vi "Motor Initial 2(SubVI).vi"(11 "Cluster in 2":T1 {"Motor Step" items=["1 deg"=1, "3 deg"=3, "5 deg"=5, "10 deg"=10]; "Motor Range" items=["40 deg"=40, "360 deg"=360, "180 deg"=180]; "Mode" items=["Create", "Delete", "Select"]; "IF Bandwidth" format="%.3p"; "Span Freq" format="%.3p"; "Center Freq" format="%.3p"; "Power Level" format="%.2p"}) -> (2 "Locat":dbl caption="Current Location" format="%#.1f deg.", 3 "Cluster in 3":T1 {"Motor Step" items=["1 deg"=1, "3 deg"=3, "5 deg"=5, "10 deg"=10]; "Motor Range" items=["40 deg"=40, "360 deg"=360, "180 deg"=180]; "Mode" items=["Create", "Delete", "Select"]; "IF Bandwidth" format="%.3p"; "Span Freq" format="%.3p"; "Center Freq" format="%.3p"; "Power Level" format="%.2p"})   [LabVIEW 2020]
uses:
  Chamber_2018/ControlCluster.ctl
  D:/BWant RT/BWant_RT.lvlibp/Control Function.ctl
  D:/BWant RT/BWant_RT.lvlibp
panel:
  in  "Stop":bool
  out "[ALM-A]":bool
  in  "Mode":enum16{"INC", "ABS"}(ring)=enum."ABS"
  out "[READY]":bool
  # "Hz"
  # "Hz"
  # "Hz"
  # "dBm"
  # "Hz"
  # "Hz"
  # "Hz"
  # "dBm"
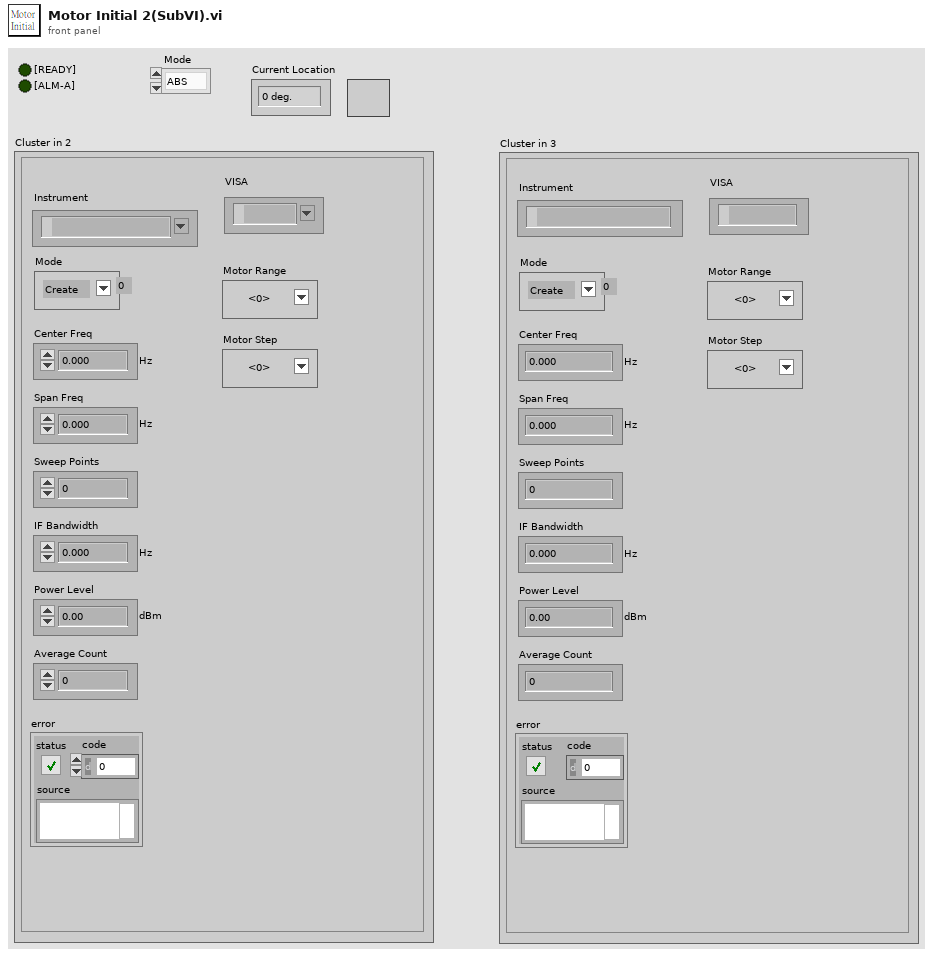
[diagram p1: front panel]
types:
  T1 = typedef "ControlCluster.ctl" = cluster{"Power Level":dbl, "Center Freq":dbl, "Span Freq":dbl, "Sweep Points":u32, "IF Bandwidth":dbl, "Average Count":i32, "error":errorcluster, "Instrument":refnum<visa-resource-name>, "Mode":u16, "Motor Range":u16, "Motor Step":u16, "VISA":refnum<visa-resource-name>}
  T2 = typedef "BWant_RT.lvlibp/Control Function.ctl" = enum16{"Idle", "Initial", "Close", "Check State", "ALM Reset", "ALM Inf", "Preset Home", "Pst_Value", "Speed", "Start-slope", "End-slpoe", "Read Pst", "GO Home", "Move", "Stop", "Limit mode", "MLU", "MLL", "Direction"}
  T3 = cluster{"[MOVE]":bool, "[READY]":bool, "[ALM-A]":bool}
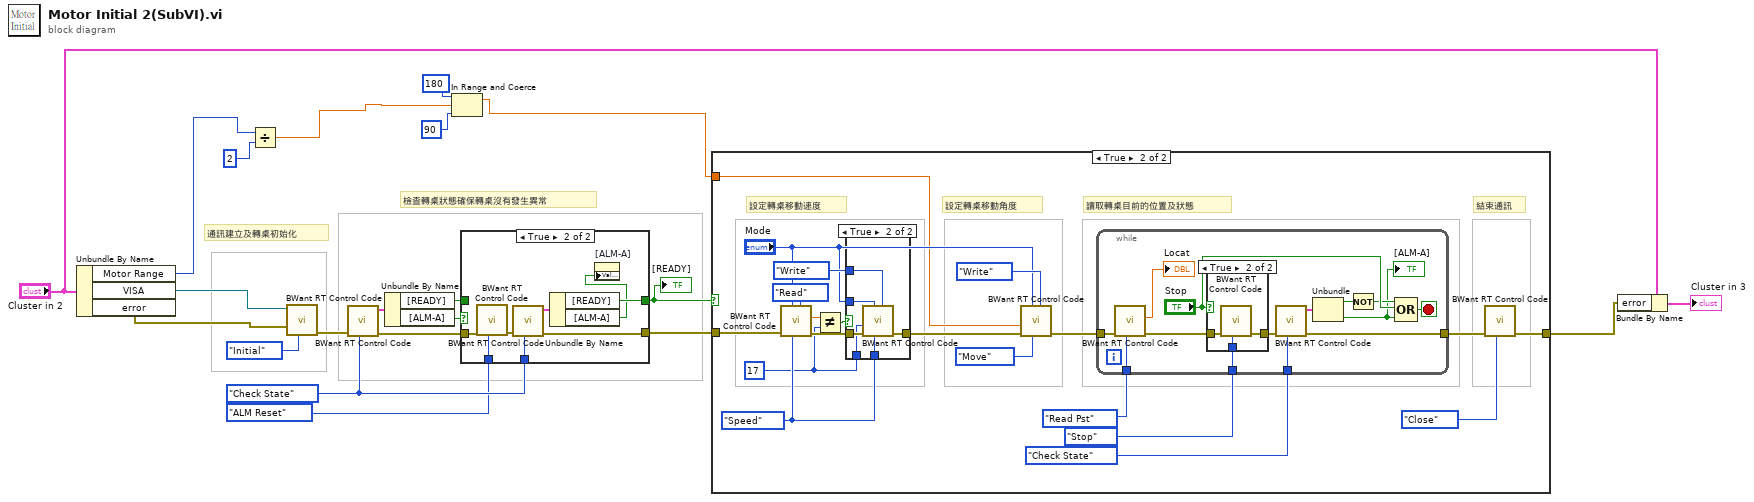
[diagram p0: block diagram]
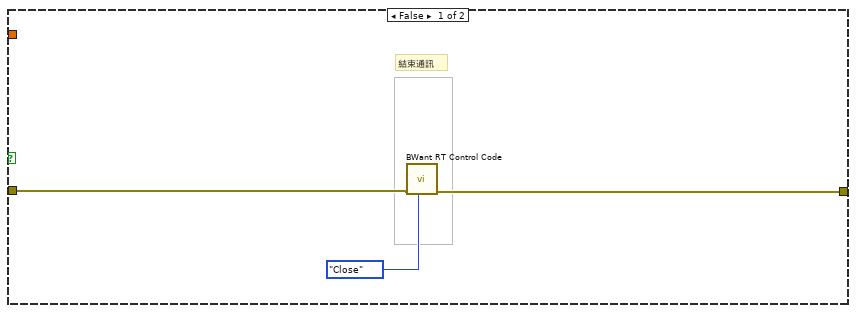
[diagram p2: hidden frame]
diagram:
  w13 = Control_Function."Check State" ("Fn")
  # "檢查轉桌狀態確保轉桌沒有發生異常"
  # "通訊建立及轉桌初始化"
  n1 = Unbundle By Name("Cluster in 2") -> ("Motor Range"=w9:u16, "VISA"=w11:refnum<visa-resource-name>, "error"=w10:errorcluster)
  n2 = Divide(x=w9, y=2) -> (x/y=w2:dbl)
  n3 = call "BWant RT Control Code.vi"("Fn"=Control_Function."Initial", "error in"=w10, "ComPort"=w11) -> ("error out"=w18:errorcluster)  [unwired: 5 in, 3 out]
  n4 = call "BWant RT Control Code.vi"("Fn"=w13, "error in"=w18) -> ("error out"=w20:errorcluster, "State"=w19:T3)  [unwired: 6 in, 2 out]
  n5 = Unbundle By Name(w19) -> ("[READY]"=w17:bool, "[ALM-A]"=w21:bool)
  n6 = In Range and Coerce(upper limit=180, x=w2, lower limit=90) -> (coerced(x)=w1:dbl)  [unwired: 1 out]
  n7 = case shown="True" w21 {
    tunnel: [w23 w29] -> w16
    tunnel: w20 -> [w23 w25]
    tunnel: Control_Function."ALM Reset" ("Fn") -> [_ w31]
    tunnel: w13 -> [_ w28]
    tunnel: [w22 w26] -> w15
    tunnel: w17 -> [w22 _]
    frame False {
    }
    frame True {
      n8 = call "BWant RT Control Code.vi"("Fn"=w31, "error in"=w25) -> ("error out"=w30:errorcluster)  [unwired: 6 in, 3 out]
      n9 = call "BWant RT Control Code.vi"("Fn"=w28, "error in"=w30) -> ("error out"=w29:errorcluster, "State"=w27:T3)  [unwired: 6 in, 2 out]
      n10 = Unbundle By Name(w27) -> ("[READY]"=w26:bool, "[ALM-A]"=w24:bool)
      n11 = property on="[ALM-A]" class="Bool (strict)"("Value"=w24) -> ()  [unwired: 2 in, 2 out]
    }
  }
  "[READY]" <- w15
  n12 = case shown="True" w15 {
    tunnel: w16 -> [w34 w54]
    tunnel: [w33 w44] -> w5
    tunnel: w1 -> [_ w36]
    frame False {
      # "結束通訊"
      n13 = call "BWant RT Control Code.vi"("Fn"=Control_Function."Close", "error in"=w34) -> ("error out"=w33:errorcluster)  [unwired: 6 in, 3 out]
    }
    frame True {
      w35 = 17
      w42 = Control_Function."Speed" ("Fn")
      # "結束通訊"
      # "讀取轉桌目前的位置及狀態"
      # "設定轉桌移動角度"
      # "設定轉桌移動速度"
      n14 = call "BWant RT Control Code.vi"("Value_RW"=enum16{"Read", "Write"}."Read", "Fn"=w42, "Mode"="Mode", "error in"=w54) -> ("error out"=w52:errorcluster, "Value out"=w51:dbl)  [unwired: 4 in, 2 out]
      n15 = Not Equal?(x=w51, y=w35) -> (x != y?=w49:bool)
      n16 = case shown="True" w49 {
        tunnel: w52 -> [w73 w79]
        tunnel: w42 -> [_ w78]
        tunnel: w35 -> [_ w77]
        tunnel: enum16{"Read", "Write"}."Write" ("Value_RW") -> [_ w76]
        tunnel: [w73 w75] -> w47
        tunnel: "Mode" -> [_ w74]
        frame False {
        }
        frame True {
          n17 = call "BWant RT Control Code.vi"("Value_RW"=w76, "Fn"=w78, "Mode"=w74, "error in"=w79, "Value in"=w77) -> ("error out"=w75:errorcluster)  [unwired: 3 in, 3 out]
        }
      }
      n18 = call "BWant RT Control Code.vi"("Value_RW"=enum16{"Read", "Write"}."Write", "Fn"=Control_Function."Move", "Mode"="Mode", "error in"=w47, "Value in"=w36) -> ("error out"=w46:errorcluster)  [unwired: 3 in, 3 out]
      n19 = while {
        tunnel: w46 -> [w68]
        tunnel: Control_Function."Read Pst" ("Fn") -> [w67]
        tunnel: Control_Function."Stop" ("Fn") -> [w64]
        tunnel: Control_Function."Check State" ("Fn") -> [w62]
        tunnel: [w60] -> w45
        stop <- w56 stop-if-true
        n20 = call "BWant RT Control Code.vi"("Fn"=w67, "error in"=w68) -> ("error out"=w65:errorcluster, "Value out"=→"Locat":dbl)  [unwired: 6 in, 2 out]
        n21 = case shown="True" "Stop" {
          tunnel: w65 -> [w69 w72]
          tunnel: w64 -> [_ w71]
          tunnel: [w69 w70] -> w63
          frame False {
          }
          frame True {
            n22 = call "BWant RT Control Code.vi"("Fn"=w71, "error in"=w72) -> ("error out"=w70:errorcluster)  [unwired: 6 in, 3 out]
          }
        }
        n23 = call "BWant RT Control Code.vi"("Fn"=w62, "error in"=w63) -> ("error out"=w60:errorcluster, "State"=w61:T3)  [unwired: 6 in, 2 out]
        n24 = Unbundle(w61) -> ("[MOVE]"=w59:bool, "[ALM-A]"=w55:bool)  [unwired: 1 out]
        "[ALM-A]" <- w55
        n25 = Not(x=w59) -> (.not. x?=w57:bool)
        n26 = Compound Arithmetic op=OR(w57, "Stop", w55) -> (w56:bool)
      }
      n27 = call "BWant RT Control Code.vi"("Fn"=Control_Function."Close", "error in"=w45) -> ("error out"=w44:errorcluster)  [unwired: 6 in, 3 out]
    }
  }
  n28 = Bundle By Name(cluster="Cluster in 2", "error"=w5) -> (→"Cluster in 3":T1)
